vi "Never Ignore Inputs.vi"(8 "error in (no error)":errorcluster, 11 "Mock in":refnum<class "LMock Mock.lvclass">) -> (0 "error out":errorcluster, 3 "Mock out":refnum<class "LMock Mock.lvclass">)   [LabVIEW 2020, in "Never.lvlib"]
uses:
  Never.lvlib
  Framework/Mock/LMock Mock.lvclass
  Comparators/Any Inputs Comparator/Any Inputs Comparator.lvclass
  C:/git/astemes-lmock/source/Core/Comparator/Comparator.lvclass
  Never.lvclass
  C:/git/astemes-lmock/source/Core/Expectation/Expectation.lvclass
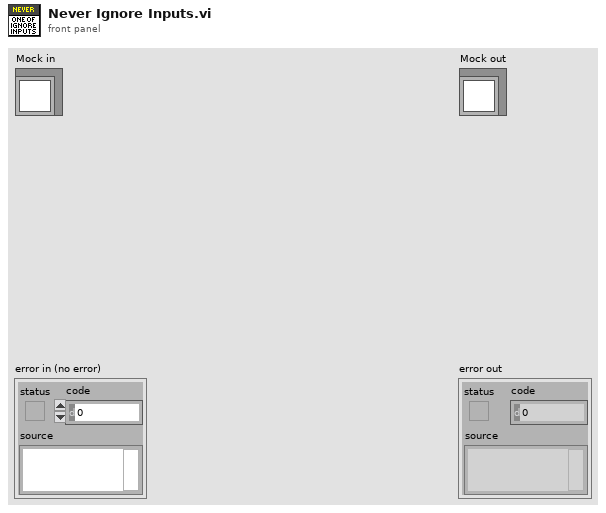
[diagram p1: front panel]
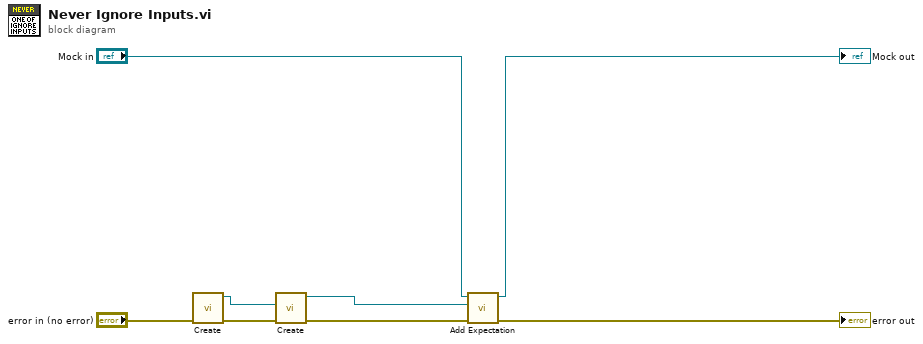
[diagram p0: block diagram]
diagram:
  n1 = call "Create.vi"("error in (no error)"="error in (no error)") -> ("error out"=w1:errorcluster, "Ignore Inputs Comparator"=w3:refnum<class "Any Inputs Comparator.lvclass">)  [unwired: 9 in]
  n2 = call "Create.vi"("error in (no error)"=w1, "Comparator"=w3) -> ("error out"=w5:errorcluster, "Never Out"=w4:refnum<class "Never.lvclass">)  [unwired: 8 in]
  n3 = call-dynamic "Add Expectation.vi"("error in (no error)"=w5, "Expectations"=w4, "Mock in"="Mock in") -> ("error out"=→"error out":errorcluster, "Mock out"=→"Mock out":refnum<class "LMock Mock.lvclass">)  [unwired: 7 in]
